vi "Enqueue-actions.vi"(7 "Enqueue mode":T3, 8 "error in (no error)":errorcluster, 9 "Timeout (ms)":i32=-1, 10 "State array":T2[](array[typedef]), 11 "State queue in":T1) -> (0 "error out":errorcluster, 1 "Timed out?":bool, 3 "State queue out":T1)   [LabVIEW 2013, in "SLMControl.lvlib" / "SC-Main.lvclass"]
doc: "Use this template to build a VI to use as a subVI."
uses:
  SC-Main.lvclass
  Enqueue-modes.ctl
  Main-actions.ctl
  Object-reference.ctl
  SC-Main.lvclass/SC-Main.ctl
  Read Action queue.vi
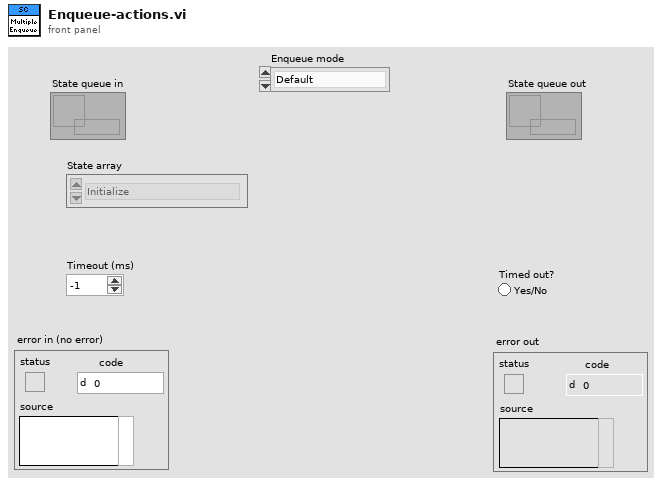
[diagram p1: front panel]
types:
  T1 = typedef "SLMControl.lvlib/SC-Main.lvclass/Object-reference.ctl" = refnum<data-value>
  T2 = typedef "SLMControl.lvlib/SC-Main.lvclass/Main-actions.ctl" = enum16{"Idle", "Initialize", "Load configuration", "Save configuration", "Load lasing files", "Load deposition files", "Refresh files", "Clear files", "Open lasing file", "Activate", "Start", "Start deposition cycle", "Start lasing cycle", "Iterate", "Abort", "Stop", "Exit"}
  T3 = typedef "SLMControl.lvlib/SC-Main.lvclass/Enqueue-modes.ctl" = enum16{"Default", "Priority", "Flush"}
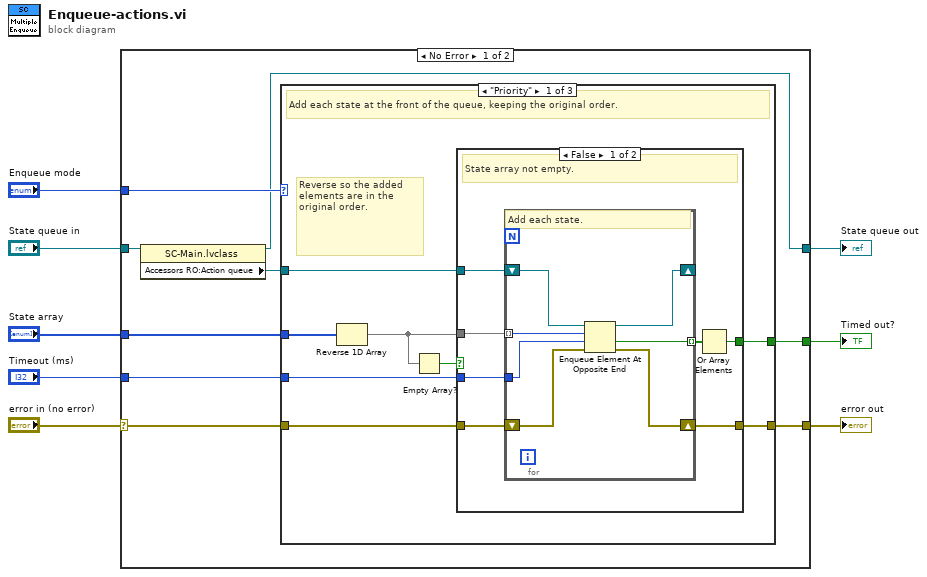
[diagram p0: block diagram]
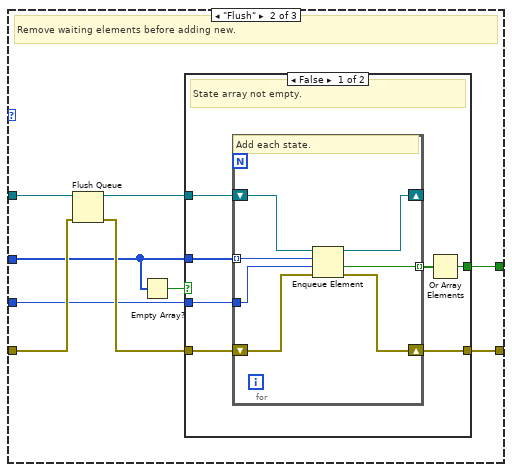
[diagram p3: hidden frame]
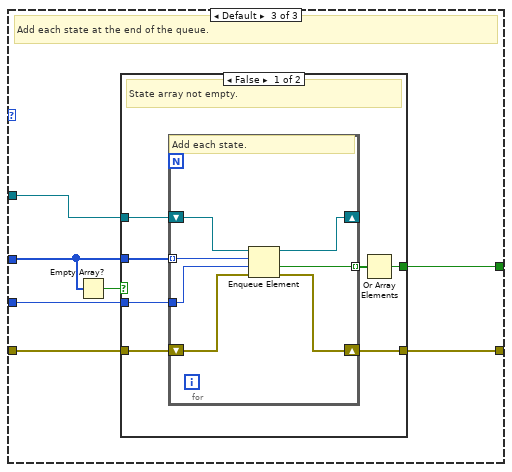
[diagram p5: hidden frame]
diagram:
  n1 = case shown="No Error" "error in (no error)" {
    selector: "error in (no error)" -> [w14 w88]
    tunnel: [w13 w88] -> w7
    tunnel: "Enqueue mode" -> [w17 _]
    tunnel: "State array" -> [w16 _]
    tunnel: "State queue in" -> [w15 w87]
    tunnel: [w9 w87] -> w3
    tunnel: "Timeout (ms)" -> [w12 _]
    tunnel: [w11 _] -> w1
    frame No Error {
      n2 = property class="SC-Main.lvclass"(reference=w15) -> (reference out=w9:T1, "Accessors RO:Action queue"=w10:refnum<queue>)  [unwired: 1 in, 1 out]
      n3 = case shown="\"Priority\"" w17 {
        tunnel: w16 -> [w25 w45 w67]
        tunnel: w10 -> [w22 w49 w70]
        tunnel: w14 -> [w21 w48 w69]
        tunnel: [w20 w42 w71] -> w13
        tunnel: w12 -> [w19 w44 w66]
        tunnel: [w18 w41 w65] -> w11
        frame "Priority" {
          # "Reverse so the added\nelements are in the original order."
          # "Add each state at the front of the queue, keeping the original order."
          n4 = Reverse 1D Array(array=w25) -> (reversed array=w23:T2[])
          n5 = Empty Array?(array=w23) -> (empty?=w24:bool)
          n6 = case shown="False" w24 {
            tunnel: [w32 w40] -> w20
            tunnel: w22 -> [w31 _]
            tunnel: w21 -> [w30 w40]
            tunnel: w23 -> [w29 _]
            tunnel: w19 -> [w28 _]
            tunnel: [w26 _] -> w18
            frame False {
              # "State array not empty."
              n7 = for {
                shift-right: [w38] -> w32
                shift-left: w30 -> [w39]
                tunnel: w29 -> [w36] mode=indexing
                shift-right: [w35] -> _
                shift-left: w31 -> [w37]
                tunnel: w28 -> [w34]
                tunnel: [w33] -> w27 mode=indexing
                # "Add each state."
                n8 = Enqueue Element At Opposite End(queue=w37, element=w36, timeout in ms (-1)=w34, error in (no error)=w39) -> (queue out=w35:refnum<queue>, timed out?=w33:bool, error out=w38:errorcluster)
              }
              n9 = Or Array Elements(Boolean array=w27) -> (logical OR=w26:bool)
            }
            frame True {
              # "Empty state array, do nothing."
            }
          }
        }
        frame "Flush" {
          # "Remove waiting elements before adding new."
          n10 = Flush Queue(queue=w49, error in (no error)=w48) -> (queue out=w43:refnum<queue>, error out=w46:errorcluster)  [unwired: 1 out]
          n11 = Empty Array?(array=w45) -> (empty?=w47:bool)
          n12 = case shown="False" w47 {
            tunnel: [w56 w64] -> w42
            tunnel: w43 -> [w55 _]
            tunnel: w46 -> [w54 w64]
            tunnel: w45 -> [w53 _]
            tunnel: w44 -> [w52 _]
            tunnel: [w50 _] -> w41
            frame False {
              # "State array not empty."
              n13 = for {
                shift-right: [w62] -> w56
                shift-left: w54 -> [w63]
                tunnel: w53 -> [w60] mode=indexing
                shift-right: [w59] -> _
                shift-left: w55 -> [w61]
                tunnel: w52 -> [w58]
                tunnel: [w57] -> w51 mode=indexing
                # "Add each state."
                n14 = Enqueue Element(queue=w61, element=w60, timeout in ms (-1)=w58, error in (no error)=w63) -> (queue out=w59:refnum<queue>, timed out?=w57:bool, error out=w62:errorcluster)
              }
              n15 = Or Array Elements(Boolean array=w51) -> (logical OR=w50:bool)
            }
            frame True {
              # "Empty state array, do nothing."
            }
          }
        }
        frame Default {
          # "Add each state at the end of the queue."
          n16 = Empty Array?(array=w67) -> (empty?=w68:bool)
          n17 = case shown="False" w68 {
            tunnel: [w78 w86] -> w71
            tunnel: w70 -> [w77 _]
            tunnel: w69 -> [w76 w86]
            tunnel: w67 -> [w75 _]
            tunnel: w66 -> [w74 _]
            tunnel: [w72 _] -> w65
            frame False {
              # "State array not empty."
              n18 = for {
                shift-right: [w84] -> w78
                shift-left: w76 -> [w85]
                tunnel: w75 -> [w82] mode=indexing
                shift-right: [w81] -> _
                shift-left: w77 -> [w83]
                tunnel: w74 -> [w80]
                tunnel: [w79] -> w73 mode=indexing
                # "Add each state."
                n19 = Enqueue Element(queue=w83, element=w82, timeout in ms (-1)=w80, error in (no error)=w85) -> (queue out=w81:refnum<queue>, timed out?=w79:bool, error out=w84:errorcluster)
              }
              n20 = Or Array Elements(Boolean array=w73) -> (logical OR=w72:bool)
            }
            frame True {
              # "Empty state array, do nothing."
            }
          }
        }
      }
    }
    frame Error {
    }
  }
  "error out" <- w7
  "State queue out" <- w3
  "Timed out?" <- w1
